vi "Keithley_Output_to_Strings.vi"(4 "Delimiter (tab)":u16(ring) items=["Tab", "New Line", "Space"], 7 "Data Format (exponential)":u16(ring)=2 items=["Float", "Integer", "Exponential"], 9 "Precision (6)":dbl=6.0, 11 "1D Array":dbl[](array[numeric])) -> (2 "String Ch 2":string, 3 "String Ch 1":string)   [LabVIEW 2013]
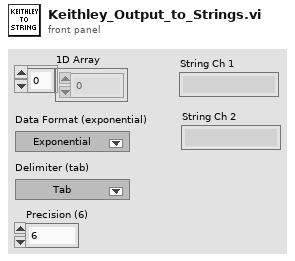
[diagram p1: front panel]
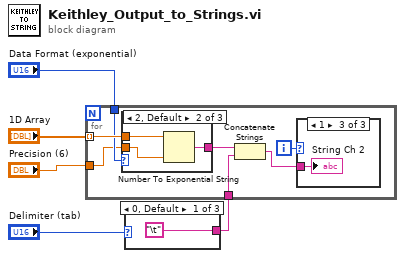
[diagram p0: block diagram]
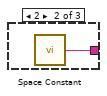
[diagram p2: hidden frame]
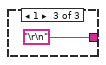
[diagram p3: hidden frame]
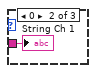
[diagram p5: hidden frame]
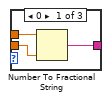
[diagram p6: hidden frame]
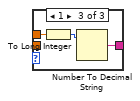
[diagram p7: hidden frame]
diagram:
  n1 = case shown="0, Default" "Delimiter (tab)" {
    tunnel: ["\t" w7 "\r\n"] -> w2
    frame 0, Default {
    }
    frame 2 {
      n2 = call <vilib>:"Space Constant.vi"() -> ("String"=w7:string)
    }
    frame 1 {
    }
  }
  n3 = for {
    tunnel: "1D Array" -> [w15] mode=indexing
    tunnel: "Data Format (exponential)" -> [w13]
    tunnel: w2 -> [w12]
    tunnel: "Precision (6)" -> [w11]
    i -> [w10]
    n4 = case shown="2, Default" w13 {
      tunnel: w15 -> [w20 w23 w26]
      tunnel: [w19 w22 w24] -> w14
      tunnel: w11 -> [w18 w21 _]
      frame 0 {
        n5 = Number To Fractional String(number=w20, precision (6)=w18) -> (F-format string=w19:string)  [unwired: 2 in]
      }
      frame 2, Default {
        n6 = Number To Exponential String(number=w23, precision (6)=w21) -> (E-format string=w22:string)  [unwired: 2 in]
      }
      frame 1 {
        n7 = To Long Integer(number=w26) -> (32bit integer=w25:i32)
        n8 = Number To Decimal String(number=w25) -> (decimal integer string=w24:string)  [unwired: 1 in]
      }
    }
    n9 = Concatenate Strings(w14, w12) -> (w9:string)
    n10 = case shown="1" w10 {
      tunnel: w9 -> [_ w16 w17]
      frame 2, Default {
      }
      frame 0 {
        "String Ch 1" <- w16
      }
      frame 1 {
        "String Ch 2" <- w17
      }
    }
  }
